vi "Joints3D.vi"() -> ()   [LabVIEW 2020]
uses:
  <vilib>/Native 3D Graph/xcontrol/3DPC_SurfacePlot.xctl
panel:
  out "3D Graph":refnum<class "Base Datatype.lvclass">[](xcontrol)
  in  "Shoulder Size 2":dbl
  in  "Shoulder Size":dbl
  in  "4 joint":dbl(slide) scale=0.0..180.0
  in  "3 joint":dbl(slide) scale=0.0..180.0
  in  "2 joint":dbl(slide) scale=0.0..180.0
  in  "1 joint":dbl(slide) scale=0.0..180.0
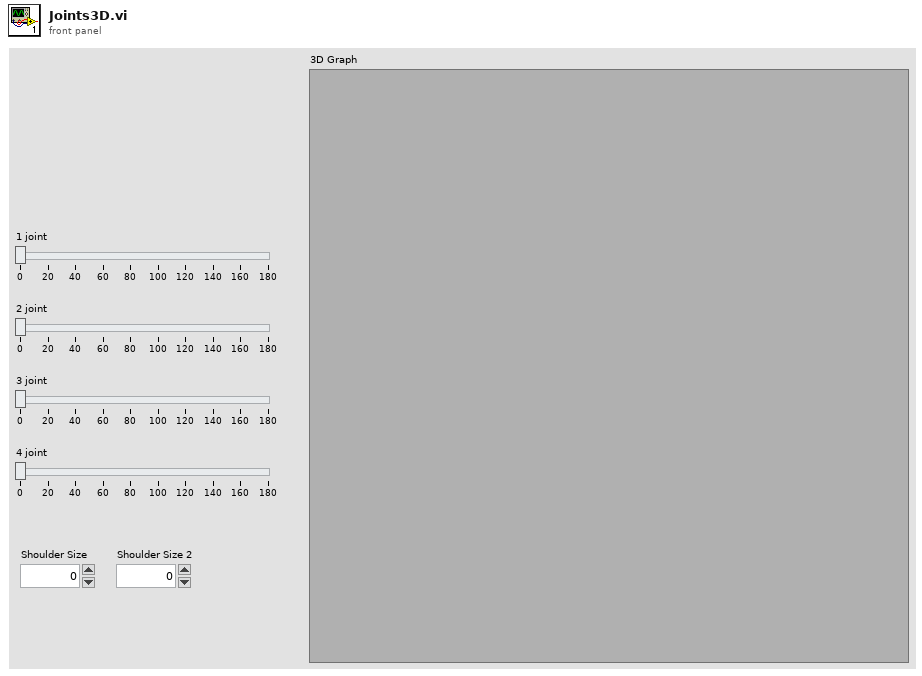
[diagram p1: front panel]
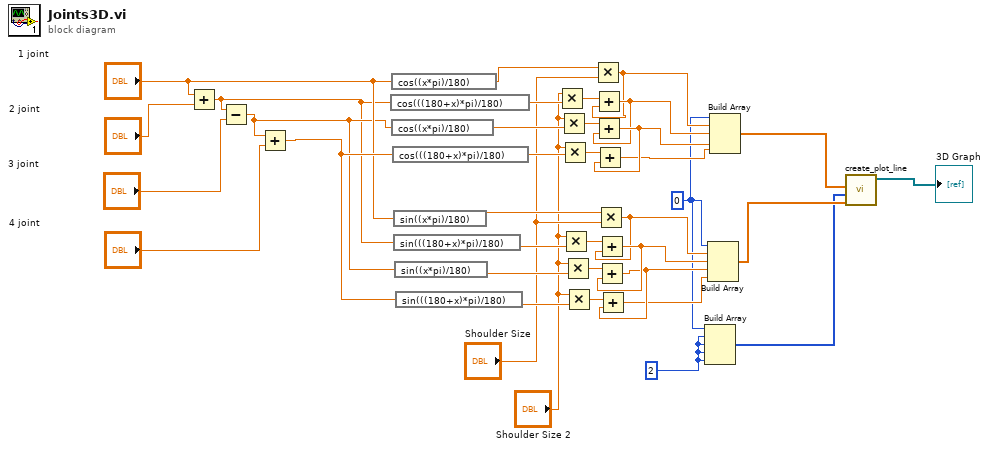
[diagram p0: block diagram]
diagram:
  w5 = 2
  w6 = 0
  n1 = Add(x="1 joint", y="2 joint") -> (x+y=w26:dbl)
  n2 = Subtract(x=w26, y="3 joint") -> (x-y=w27:dbl)
  n3 = Add(x=w27, y="4 joint") -> (x+y=w29:dbl)
  n4 = expression code="cos(((180+x)*pi)/180)"(w26) -> (w22:dbl)
  n5 = expression code="cos((x*pi)/180)"("1 joint") -> (w37:dbl)
  n6 = expression code="cos((x*pi)/180)"(w27) -> (w17:dbl)
  n7 = expression code="cos(((180+x)*pi)/180)"(w29) -> (w18:dbl)
  n8 = expression code="sin((x*pi)/180)"("1 joint") -> (w36:dbl)
  n9 = expression code="sin(((180+x)*pi)/180)"(w26) -> (w20:dbl)
  n10 = expression code="sin((x*pi)/180)"(w27) -> (w13:dbl)
  n11 = expression code="sin(((180+x)*pi)/180)"(w29) -> (w12:dbl)
  n12 = Multiply(x="Shoulder Size 2", y=w22) -> (x*y=w23:dbl)
  n13 = Multiply(x="Shoulder Size 2", y=w17) -> (x*y=w19:dbl)
  n14 = Multiply(x="Shoulder Size 2", y=w18) -> (x*y=w16:dbl)
  n15 = Multiply(x="Shoulder Size 2", y=w20) -> (x*y=w21:dbl)
  n16 = Multiply(x="Shoulder Size 2", y=w13) -> (x*y=w14:dbl)
  n17 = Multiply(x="Shoulder Size 2", y=w12) -> (x*y=w15:dbl)
  n18 = Multiply(x=w37, y="Shoulder Size") -> (x*y=w25:dbl)
  n19 = Add(x=w23, y=w25) -> (x+y=w34:dbl)
  n20 = Add(x=w19, y=w34) -> (x+y=w35:dbl)
  n21 = Add(x=w16, y=w35) -> (x+y=w33:dbl)
  n22 = Multiply(x=w36, y="Shoulder Size") -> (x*y=w24:dbl)
  n23 = Add(x=w21, y=w24) -> (x+y=w32:dbl)
  n24 = Add(x=w14, y=w32) -> (x+y=w31:dbl)
  n25 = Add(x=w15, y=w31) -> (x+y=w30:dbl)
  n26 = Build Array(w6, w5, w5, w5, w5) -> (w2:i32[])
  n27 = Build Array(w6, w24, w32, w31, w30) -> (w3:dbl[])
  n28 = Build Array(w6, w25, w34, w35, w33) -> (w1:dbl[])
  n29 = call <vilib>:"create_plot_line.vi"("z vector"=w3, "y vector"=w2, "x vector"=w1) -> ("plots out"=→"3D Graph":refnum<class "Base Datatype.lvclass">[])  [unwired: 2 in, 6 out]
